vi "LickSpout_VolumeTest.vi"() -> ()   [LabVIEW 2019]
doc: "The myRIO Project template acquires acceleration data from the onboard accelerometer and displays the changes of acceleration values in a waveform chart."
uses:
  <vilib>/myRIO/Common/Instrument Driver Framework/Utilities/typedefs/Generic FPGA Reference.ctl
  <vilib>/myRIO/Common/Instrument Driver Framework/Utilities/typedefs/myRIO v1.0 Reference.ctl
  <vilib>/myRIO/Common/Instrument Driver Framework/Utilities/typedefs/Hardware Version Enum.ctl
  <vilib>/myRIO/Common/Instrument Driver Framework/Utilities/typedefs/myRIO Generic Hardware Reference.ctl
  <vilib>/userdefined/High Color/nirio_resource_hc.ctl
  <vilib>/myRIO/Common/Instrument Driver Framework/Utilities/vis/Is FPGA Ref Available.vi
  <vilib>/myRIO/Common/Instrument Driver Framework/myRIO v1.0/Encoder/typedefs/Encoder Signal Mode.ctl
  <vilib>/myRIO/Common/Instrument Driver Framework/myRIO v1.0/Encoder/typedefs/Encoder Channels Enum.ctl
  <vilib>/myRIO/Instrument Drivers/Onboard IO/Encoder/typedefs/Encoder Reference.ctl
  <vilib>/myRIO/Instrument Drivers/Onboard IO/Encoder/Encoder.lvlib
  <vilib>/myRIO/Instrument Drivers/Onboard IO/Encoder/vis/Read.vi
  <vilib>/myRIO/Common/Instrument Driver Framework/myRIO v1.0/Encoder/typedefs/Encoder Configuration v1.0.ctl
  <vilib>/myRIO/Common/Instrument Driver Framework/myRIO v1.0/Encoder/vis/myRIO v1.1 Open Encoder.vi
  <vilib>/myRIO/Common/Instrument Driver Framework/myRIO v1.0/Encoder/vis/myRIO v1.0 Configure Encoder.vi
  <vilib>/myRIO/Instrument Drivers/Onboard IO/Encoder/vis/myRIO Encoder Open.xnode
  <vilib>/myRIO/Express VI/Onboard IO/Encoder/Encoder Express VI.xnode
  <vilib>/myRIO/Express VI/Onboard IO/DI/DI Express VI.xnode
  <vilib>/myRIO/Instrument Drivers/Onboard IO/DIO/vis/Read.vi
  <vilib>/myRIO/Instrument Drivers/Onboard IO/DIO/DIO.lvlib
  <vilib>/myRIO/Common/Instrument Driver Framework/myRIO v1.0/DIO/typedefs/DIO Channels Enum.ctl
  <vilib>/myRIO/Common/Instrument Driver Framework/myRIO v1.0/DIO/typedefs/DIO Channels List.ctl
  <vilib>/myRIO/Instrument Drivers/Onboard IO/DIO/typedefs/DIO Reference.ctl
  <vilib>/myRIO/Instrument Drivers/Onboard IO/DIO/vis/myRIO DIO Open.xnode
  <vilib>/myRIO/Common/Instrument Driver Framework/myRIO v1.0/DIO/vis/myRIO v1.1 Open DIO.vi
  <vilib>/myRIO/Instrument Drivers/Onboard IO/DIO/vis/Write.vi
  <vilib>/myRIO/Express VI/Onboard IO/DO/DO Express VI.xnode
panel:
  out "Stop Button 3":bool
  out "MaxRewards":i32=100
  out "Speed":dbl
  in  "Stop Button":bool
  out "Time since last reward":dbl
  out "Time of last reward":dbl
  out "Rewards":u16
  out "Frame clock":i32
  out "Frames":u32
  out "Reward":bool=TRUE
  in  "Give reward":bool
  out "Licks":u32
  out "Lick":bool
  out "Output":dbl[][](array[numeric])
  out "Time":dbl
  out "Display":bool
  out "Overflow?":bool
  out "Counter Value":i32
  out "Velocity":dbl
  out "Velocity Plot":dbl[](graph)
  out "Velocity array":dbl[](array[numeric])
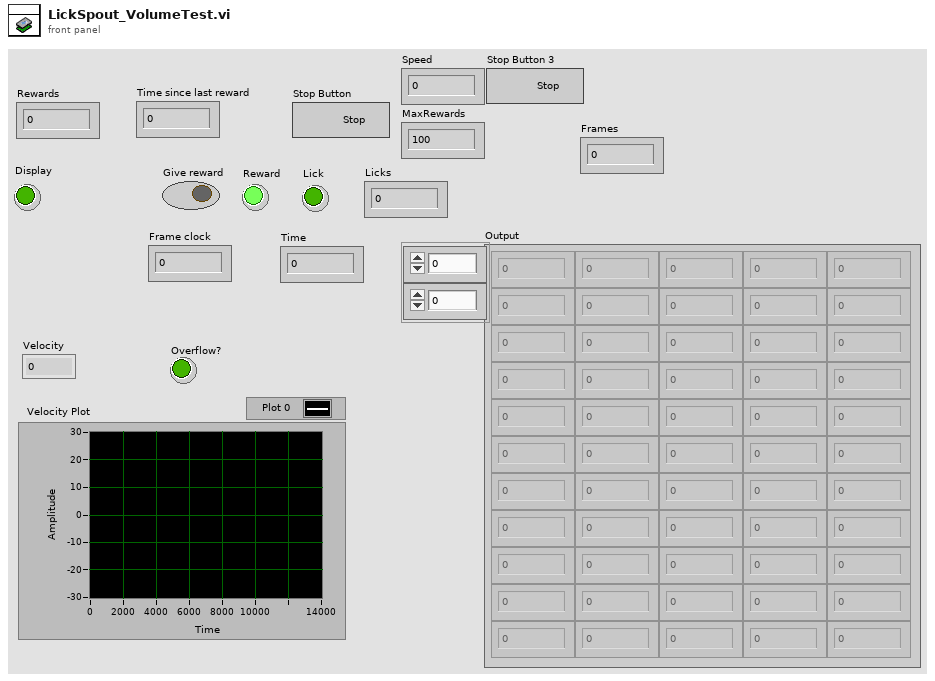
[diagram p1: front panel]
types:
  T1 = typedef "Encoder.lvlib/Encoder Reference.ctl" = cluster{"myRIO Reference":T2, "Encoder Channels Enum":T6}
  T2 = typedef "myRIO Generic Hardware Reference.ctl" = cluster{"myRIO Model":T3, "myRIO Hardware Reference":T4}
  T3 = typedef "Hardware Version Enum.ctl" = enum16{"Unknown", "myRIO-1900", "myRIO-1950", "roboRIO", "NI ELVIS RIO CM", "ELVIS III"}
  T4 = typedef "myRIO v1.0 Reference.ctl" = cluster{"Generic FPGA Reference":T5, "Allow multiple opens":bool}
  T5 = typedef "Generic FPGA Reference.ctl" = refnum<k20>
  T6 = typedef "Encoder Channels Enum.ctl" = enum16{"Not Connected", "C/ENC0", "C/ENC1", "A/ENC", "A/ENC0", "A/ENC1", "A/ENC2", "A/ENC3", "A/ENC4", "A/ENC5", "A/ENC6", "A/ENC7", "A/ENC8", "A/ENC9", "B/ENC", "B/ENC0", "B/ENC1", "B/ENC2", "B/ENC3", "B/ENC4", "B/ENC5", "B/ENC6", "B/ENC7", "B/ENC8", "B/ENC9", "DIO/ENC0", "DIO/ENC1", "DIO/ENC2", "DIO/ENC3", "DIO/ENC4"}
  T7 = typedef "Encoder Signal Mode.ctl" = enum16{"Quadrature phase signal", "Step and direction signal"}
  T8 = typedef "nirio_resource_hc.ctl" = tag
  T9 = typedef "DIO.lvlib/DIO Reference.ctl" = cluster{"myRIO Reference":T2, "DIO Channels List":T10}
  T10 = typedef "DIO Channels List.ctl" = T11[]
  T11 = typedef "DIO Channels Enum.ctl" = enum16{"Not Connected", "C/DIO0", "C/DIO1", "C/DIO2", "C/DIO3", "C/DIO4", "C/DIO5", "C/DIO6", "C/DIO7", "A/DIO0", "A/DIO1", "A/DIO2", "A/DIO3", "A/DIO4", "A/DIO5", "A/DIO6", "A/DIO7", "A/DIO8", "A/DIO9", "A/DIO10", "A/DIO11", "A/DIO12", "A/DIO13", "A/DIO14", "A/DIO15", "A/DIO16", "A/DIO17", "A/DIO18", "A/DIO19", "B/DIO0", "B/DIO1", "B/DIO2", "B/DIO3", "B/DIO4", "B/DIO5", "B/DIO6", "B/DIO7", "B/DIO8", "B/DIO9", "B/DIO10", "B/DIO11", "B/DIO12", "B/DIO13", "B/DIO14", "B/DIO15", "B/DIO16", "B/DIO17", "B/DIO18", "B/DIO19", "LED0", "LED1", "LED2", "LED3", "Button0", "DIO/DIO0", "DIO/DIO1", "DIO/DIO2", "DIO/DIO3", "DIO/DIO4", "DIO/DIO5", "DIO/DIO6", "DIO/DIO7", "DIO/DIO8", "DIO/DIO9", "SPI/CS0", "SPI/CS1", "SPI/CS2", "SPI/CS3", "LED RADIO (Green)", "LED RADIO (Red)", "LED COMM (Green)", "LED COMM (Red)", "LED MODE (Green)", "LED MODE (Red)"}
  T12 = typedef "NI_Matrix.lvlib/RealMatrix.ctl" = dbl[][]
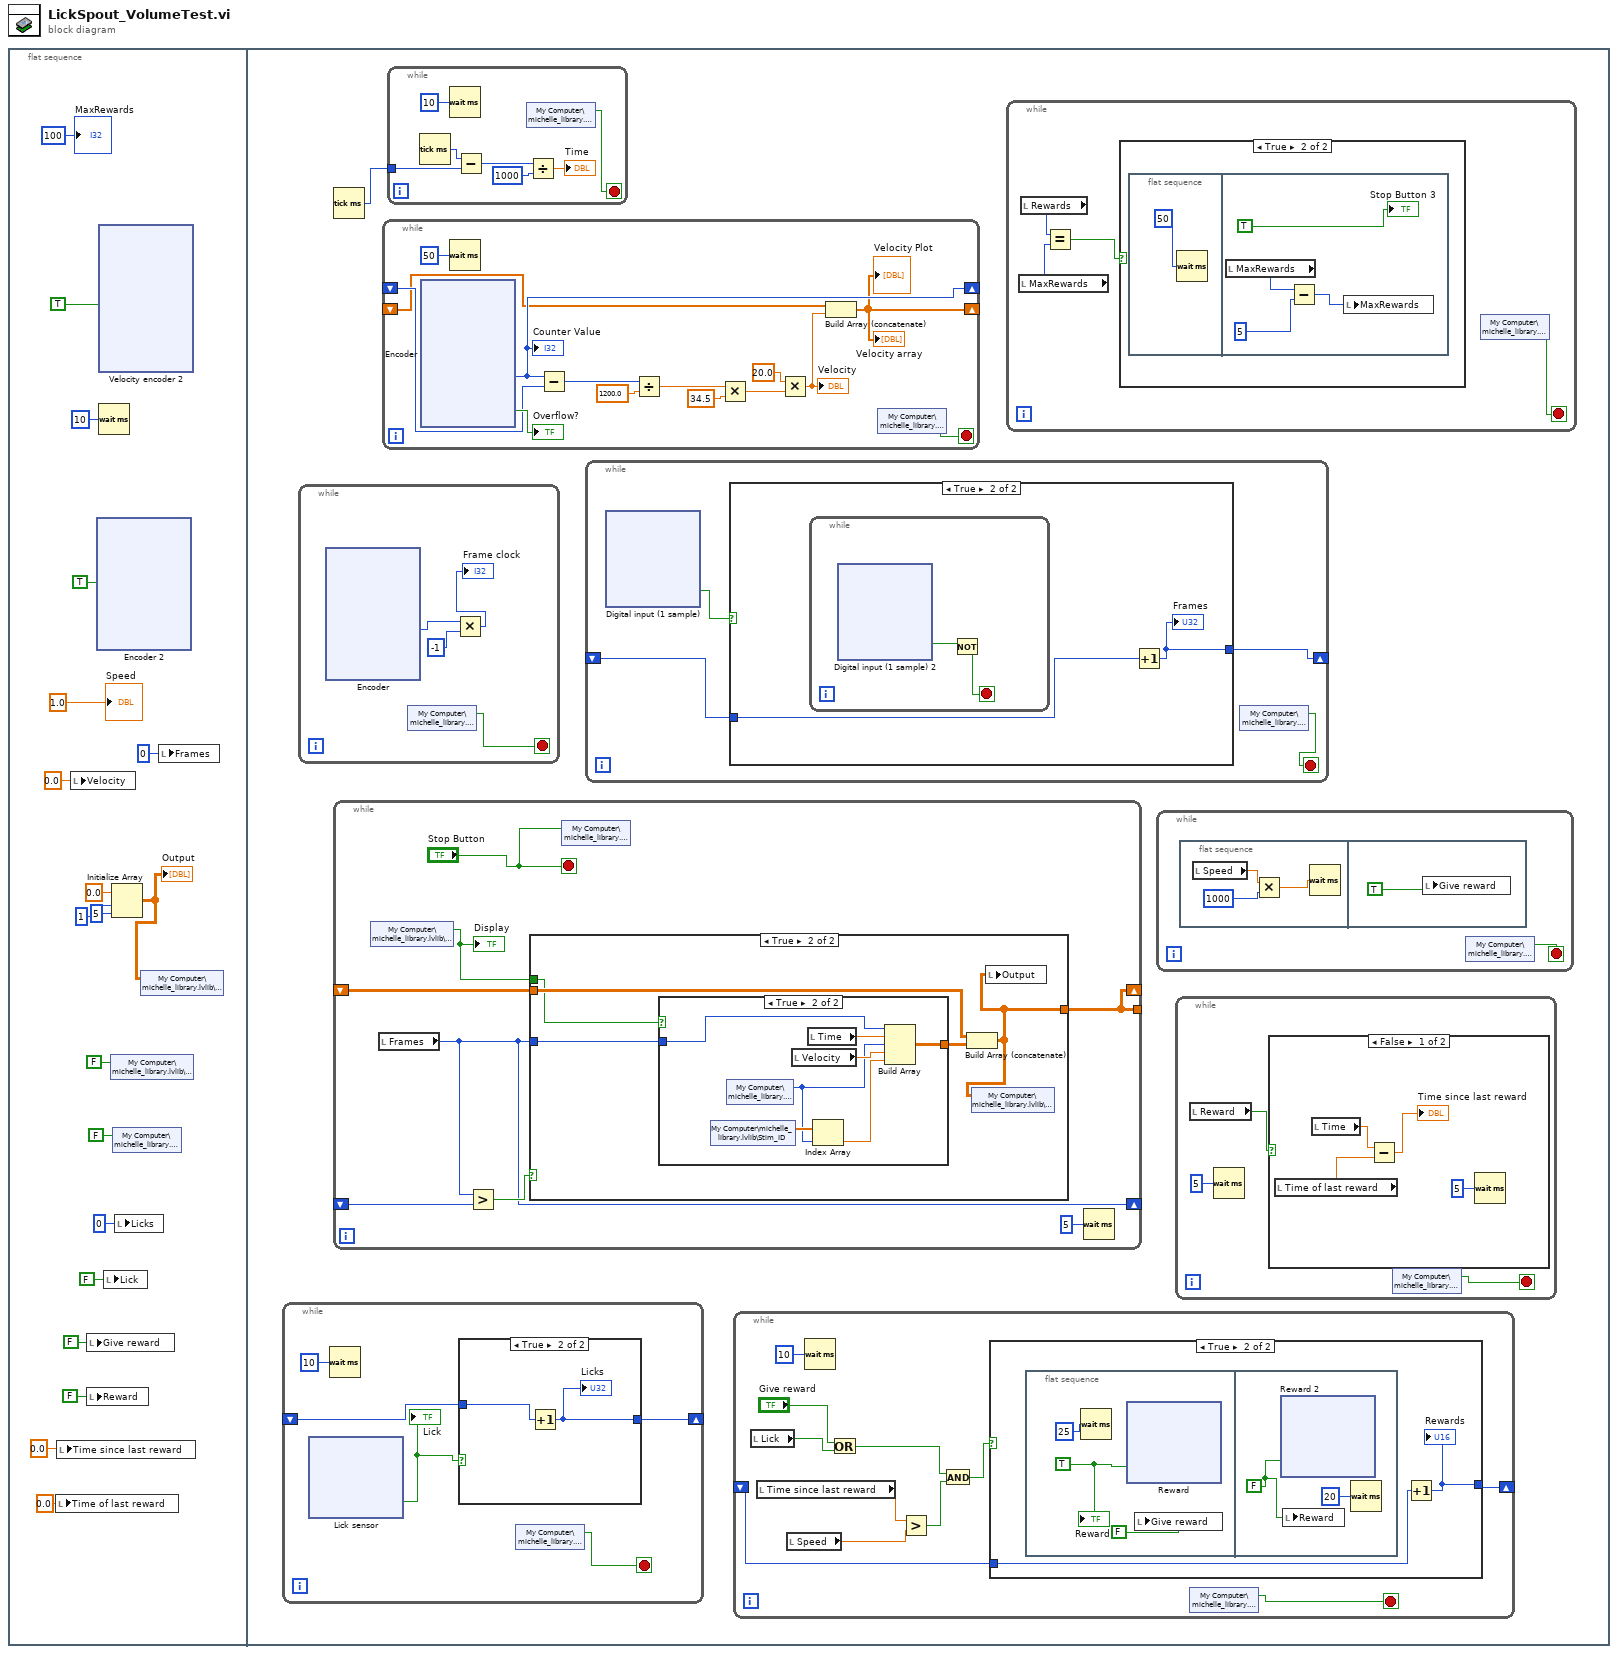
[diagram p0: block diagram]
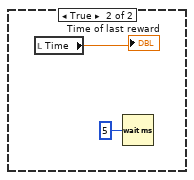
[diagram p3: hidden frame]
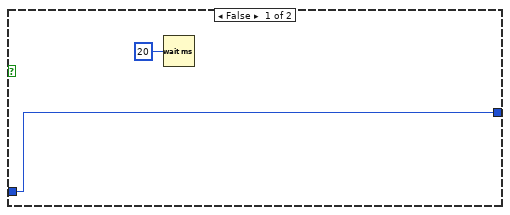
[diagram p5: hidden frame]
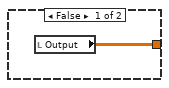
[diagram p7: hidden frame]
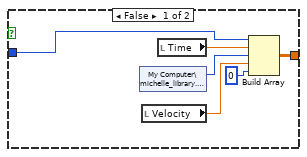
[diagram p8: hidden frame]
diagram:
  n1 = flat-sequence {
    frame #0 {
      n2 = local write "Time of last reward"(0.0 ("Time of last reward")) -> ()
      n3 = local write "Time since last reward"(0.0 ("Time since last reward")) -> ()
      n4 = local write "Velocity"(0.0 ("Velocity")) -> ()
      n5 = local write "Give reward"(FALSE ("Give reward")) -> ()
      n6 = local write "Reward"(FALSE ("Reward")) -> ()
      n7 = xnode "Encoder 2"("Reset Counter"=TRUE) -> ()  [unwired: 1 in, 4 out]
      n8 = xnode "Velocity encoder 2"("Reset Counter"=TRUE) -> ()  [unwired: 1 in, 4 out]
      n9 = Wait (ms)(milliseconds to wait=u32 10) -> ()  [unwired: 1 out]
      n10 = local write "Lick"(FALSE ("Lick")) -> ()
      n11 = shared-variable "My Computer\\michelle_library.lvlib\\Display"(FALSE ("Display")) -> ()  [unwired: 1 in, 1 out]
      n12 = Initialize Array(0.0 ("element"), 1 ("dimension size"), 5 ("dimension size")) -> (w13:dbl[][])
      "Output" <- w13
      n13 = shared-variable "My Computer\\michelle_library.lvlib\\Stop"(FALSE ("Stop")) -> ()  [unwired: 1 in, 1 out]
      n14 = local write "Licks"(u32 0 ("Licks")) -> ()
      n15 = shared-variable "My Computer\\michelle_library.lvlib\\Output"(w13) -> ()  [unwired: 1 in, 1 out]
      n16 = local write "Frames"(u32 0 ("Frames")) -> ()
      "Speed" <- 1.0
      "MaxRewards" <- 100
    }
    frame #1 {
      n17 = while {
        shift-right: [w356] -> _
        shift-left: _ -> [w355]
        stop <- w359 stop-if-true
        n18 = xnode "Lick sensor"() -> ("C/DIO1 (DIO1)"=w357:bool)  [unwired: 1 in, 1 out]
        "Lick" <- w357
        n19 = Wait (ms)(milliseconds to wait=u32 10) -> ()  [unwired: 1 out]
        n20 = case shown="True" w357 {
          tunnel: [w360 w362] -> w356
          tunnel: w355 -> [w360 w361]
          frame False {
          }
          frame True {
            n21 = Increment(x=w361) -> (x+1=w362:u32)
            "Licks" <- w362
          }
        }
        n22 = shared-variable "My Computer\\michelle_library.lvlib\\Stop"() -> (w359:bool)  [unwired: 1 in, 1 out]
      }
      n23 = while {
        stop <- w136 stop-if-true
        n24 = xnode "Encoder"() -> ("Counter Value"=w139:i32)  [unwired: 2 in, 3 out]
        n25 = shared-variable "My Computer\\michelle_library.lvlib\\Stop"() -> (w136:bool)  [unwired: 1 in, 1 out]
        n26 = Multiply(x=w139, y=-1) -> (x*y=→"Frame clock":i32)
      }
      n27 = Tick Count (ms)() -> (millisecond timer value=w112:u32)
      n28 = while {
        shift-right: [w470] -> _
        shift-left: _ -> [w472]
        shift-right: [w467] -> _
        shift-left: _ -> [w469]
        tunnel: [w467] -> _
        stop <- "Stop Button" stop-if-true
        n29 = shared-variable "My Computer\\michelle_library.lvlib\\Display"() -> (w466:bool)  [unwired: 1 in, 1 out]
        "Display" <- w466
        n30 = local read "Frames"() -> (w470:u32)
        n31 = Greater?(x=w470, y=w472) -> (0:w471:bool)
        n32 = case shown="True" w471 {
          tunnel: w470 -> [_ w478]
          tunnel: w469 -> [_ w477]
          tunnel: [w473 w474] -> w467
          tunnel: w466 -> [_ w475]
          frame False {
            n33 = local read "Output"() -> (w473:dbl[][])
          }
          frame True {
            n34 = case shown="True" w475 {
              tunnel: w478 -> [w479 w491]
              tunnel: [w483 w490] -> w476
              frame False {
                n35 = shared-variable "My Computer\\michelle_library.lvlib\\Trial"() -> (w481:u32)  [unwired: 1 in, 1 out]
                n36 = local read "Velocity"() -> (w480:dbl)
                n37 = local read "Time"() -> (w482:dbl)
                n38 = Build Array(w479, w482, w481, w480, 0) -> (w483:T12)
              }
              frame True {
                n39 = shared-variable "My Computer\\michelle_library.lvlib\\Stim_ID"() -> (w487:dbl[])  [unwired: 1 in, 1 out]
                n40 = shared-variable "My Computer\\michelle_library.lvlib\\Trial"() -> (w486:u32)  [unwired: 1 in, 1 out]
                n41 = local read "Velocity"() -> (w488:dbl)
                n42 = local read "Time"() -> (w489:dbl)
                n43 = Index Array(array=w487, index=w486) -> (element=w485:dbl)
                n44 = Build Array(w491, w489, w486, w488, w485) -> (w490:T12)
              }
            }
            n45 = Build Array (concatenate)(w477, w476) -> (w474:T12)
            n46 = shared-variable "My Computer\\michelle_library.lvlib\\Output"(w474) -> ()  [unwired: 1 in, 1 out]
            n47 = local write "Output"(w474) -> ()
          }
        }
        n48 = shared-variable "My Computer\\michelle_library.lvlib\\Stop"("Stop Button") -> ()  [unwired: 1 in, 1 out]
        n49 = Wait (ms)(milliseconds to wait=u32 5) -> ()  [unwired: 1 out]
      }
      n50 = while {
        shift-right: [w408] -> _
        shift-left: _ -> [w409]
        shift-right: [w400] -> _
        shift-left: _ -> [w399]
        stop <- w398 stop-if-true
        n51 = xnode "Encoder"() -> ("Counter Value"=w408:i32, "Overflow?"=→"Overflow?":bool)  [unwired: 2 in, 2 out]
        "Counter Value" <- w408
        n52 = Wait (ms)(milliseconds to wait=u32 50) -> ()  [unwired: 1 out]
        n53 = Subtract(x=w408, y=w409) -> (x-y=w401:i32)
        n54 = Divide(x=w401, y=1200.0 ("600")) -> (x/y=w406:dbl)
        n55 = Multiply(x=w406, y=34.5) -> (x*y=w404:dbl)
        n56 = Multiply(x=20.0, y=w404) -> (x*y=w402:dbl)
        "Velocity" <- w402
        n57 = Build Array (concatenate)(w399, w402) -> (w400:dbl[])
        "Velocity Plot" <- w400
        "Velocity array" <- w400
        n58 = shared-variable "My Computer\\michelle_library.lvlib\\Stop"() -> (w398:bool)  [unwired: 1 in, 1 out]
      }
      n59 = while {
        tunnel: w112 -> [w463]
        stop <- w458 stop-if-true
        n60 = Tick Count (ms)() -> (millisecond timer value=w464:u32)
        n61 = Wait (ms)(milliseconds to wait=u32 10) -> ()  [unwired: 1 out]
        n62 = Subtract(x=w464, y=w463) -> (x-y=w461:u32)
        n63 = shared-variable "My Computer\\michelle_library.lvlib\\Stop"() -> (w458:bool)  [unwired: 1 in, 1 out]
        n64 = Divide(x=w461, y=u32 1000) -> (x/y=→"Time":dbl)
      }
      n65 = while {
        shift-right: [w189] -> _
        shift-left: _ -> [w188]
        stop <- w187 stop-if-true
        n66 = xnode "Digital input (1 sample)"() -> ("A/DIO13 (Pin 26)"=w186:bool)  [unwired: 1 in, 1 out]
        n67 = case shown="True" w186 {
          tunnel: [w225 w227] -> w189
          tunnel: w188 -> [w225 w226]
          frame False {
          }
          frame True {
            n68 = while {
              stop <- w229 stop-if-true
              n69 = xnode "Digital input (1 sample) 2"() -> ("A/DIO13 (Pin 26)"=w228:bool)  [unwired: 1 in, 1 out]
              n70 = Not(x=w228) -> (.not. x?=w229:bool)
            }
            n71 = Increment(x=w226) -> (x+1=w227:u32)
            "Frames" <- w227
          }
        }
        n72 = shared-variable "My Computer\\michelle_library.lvlib\\Stop"() -> (w187:bool)  [unwired: 1 in, 1 out]
      }
      n73 = while {
        shift-right: [w274] -> _
        shift-left: _ -> [w273]
        stop <- w275 stop-if-true
        n74 = local read "Lick"() -> (w271:bool)
        n75 = local read "Time since last reward"() -> (w269:dbl)
        n76 = local read "Speed"() -> (w265:dbl)
        n77 = Wait (ms)(milliseconds to wait=u32 10) -> ()  [unwired: 1 out]
        n78 = Or(x="Give reward", y=w271) -> (x .or. y?=w267:bool)
        n79 = Greater?(x=w269, y=w265) -> (0:w268:bool)
        n80 = And(x=w267, y=w268) -> (x .and. y?=w266:bool)
        n81 = case shown="True" w266 {
          tunnel: [w277 w279] -> w274
          tunnel: w273 -> [w277 w278]
          frame False {
            n82 = Wait (ms)(milliseconds to wait=u32 20) -> ()  [unwired: 1 out]
          }
          frame True {
            n83 = flat-sequence {
              frame #0 {
                w282 = TRUE ("C/DIO0 (DIO0)")
                n84 = Wait (ms)(milliseconds to wait=u32 25) -> ()  [unwired: 1 out]
                n85 = xnode "Reward"("C/DIO0 (DIO0)"=w282) -> ()  [unwired: 1 in, 1 out]
                n86 = local write "Give reward"(FALSE ("Give reward")) -> ()
                "Reward" <- w282
              }
              frame #1 {
                w319 = FALSE ("C/DIO0 (DIO0)")
                n87 = xnode "Reward 2"("C/DIO0 (DIO0)"=w319) -> ()  [unwired: 1 in, 1 out]
                n88 = local write "Reward"(w319) -> ()
                n89 = Wait (ms)(milliseconds to wait=u32 20) -> ()  [unwired: 1 out]
              }
            }
            n90 = Increment(x=w278) -> (x+1=w279:u16)
            "Rewards" <- w279
          }
        }
        n91 = shared-variable "My Computer\\michelle_library.lvlib\\Stop"() -> (w275:bool)  [unwired: 1 in, 1 out]
      }
      n92 = while {
        stop <- w113 stop-if-true
        n93 = local read "MaxRewards"() -> (w115:i32)
        n94 = local read "Rewards"() -> (w116:u16)
        n95 = Equal?(x=w116, y=w115) -> (x = y?=w114:bool)
        n96 = case shown="True" w114 {
          frame False {
          }
          frame True {
            n97 = flat-sequence {
              frame #0 {
                n98 = Wait (ms)(milliseconds to wait=50) -> ()  [unwired: 1 out]
              }
              frame #1 {
                n99 = local read "MaxRewards"() -> (w121:i32)
                n100 = Subtract(x=w121, y=5) -> (x-y=w119:i32)
                n101 = local write "MaxRewards"(w119) -> ()
                "Stop Button 3" <- TRUE
              }
            }
          }
        }
        n102 = shared-variable "My Computer\\michelle_library.lvlib\\Stop"() -> (w113:bool)  [unwired: 1 in, 1 out]
      }
      n103 = while {
        stop <- w122 stop-if-true
        n104 = flat-sequence {
          frame #0 {
            n105 = local read "Speed"() -> (w124:dbl)
            n106 = Multiply(x=w124, y=1000) -> (x*y=w125:dbl)
            n107 = Wait (ms)(milliseconds to wait=w125) -> ()  [unwired: 1 out]
          }
          frame #1 {
            n108 = local write "Give reward"(TRUE) -> ()
          }
        }
        n109 = shared-variable "My Computer\\michelle_library.lvlib\\Stop"() -> (w122:bool)  [unwired: 1 in, 1 out]
      }
      n110 = while {
        stop <- w127 stop-if-true
        n111 = local read "Reward"() -> (w129:bool)
        n112 = Wait (ms)(milliseconds to wait=u32 5) -> ()  [unwired: 1 out]
        n113 = case shown="False" w129 {
          frame False {
            n114 = local read "Time of last reward"() -> (w131:dbl)
            n115 = local read "Time"() -> (w132:dbl)
            n116 = Subtract(x=w132, y=w131) -> (x-y=→"Time since last reward":dbl)
            n117 = Wait (ms)(milliseconds to wait=u32 5) -> ()  [unwired: 1 out]
          }
          frame True {
            n118 = local read "Time"() -> (→"Time of last reward":dbl)
            n119 = Wait (ms)(milliseconds to wait=u32 5) -> ()  [unwired: 1 out]
          }
        }
        n120 = shared-variable "My Computer\\michelle_library.lvlib\\Stop"() -> (w127:bool)  [unwired: 1 in, 1 out]
      }
    }
  }
